vi "d(f4+g4u)_dx3.vi"(1 "x3_":dbl, 3 "x4_":dbl, 5 "F":dbl) -> (22 "d(f4+g4u)/dx3":dbl)   [LabVIEW 2014]
uses:
  <vilib>/Simulation/Implementation/Shared/SIMSCR Execution Mode.ctl
  <vilib>/Simulation/Scripting/Companion Diagram/SimConfigNode/SimParams.ctl
  <vilib>/Simulation/Scripting/Companion Diagram/SimConfigNode/_simSolvers.ctl
  <vilib>/Simulation/Param Hierarchy/Typedefs/SIMPH Param Control Actions.ctl
  <vilib>/Simulation/Implementation/Shared/NILVSim_ParamChanged.vi
  <vilib>/Simulation/Implementation/Shared/NILVSIM_BeginStep.vi
  <vilib>/Simulation/SignalArithmetic/Implementation/NILVSim Gain.llb/SIM Gain (scalar).vi
  <vilib>/Simulation/Implementation/Shared/NILVSim_Manager.vi
  <vilib>/Utility/error.llb/Clear Errors.vi
  <vilib>/Simulation/Implementation/Shared/NILVSim_FinalizeModel.vi
  <vilib>/Simulation/Implementation/Shared/SIM Unbundle Sim Info.vi
  <vilib>/Simulation/Implementation/Shared/SIMSH Read Queue.vi
  <vilib>/Simulation/Implementation/Shared/NILVSim_Initialize.vi
  <vilib>/Simulation/Utility/Implementation/NILVSim Get Time and IsAcceptedStep.vi
  <vilib>/Simulation/Implementation/Shared/NILVSim_GetModelError.vi
  <vilib>/Simulation/Implementation/Shared/SIM SimErrorHandler.vi
  <vilib>/Simulation/Implementation/Shared/SIM Bundle Sim Info.vi
  <vilib>/Simulation/Scripting/Companion Diagram/SimConfigNode/SimDog.xnode
  <vilib>/Simulation/Implementation/XNodeFramework/SimXNode/SimX.xnode
  <vilib>/Simulation/Implementation/Shared/NI_SIM_Implementation.lvlib
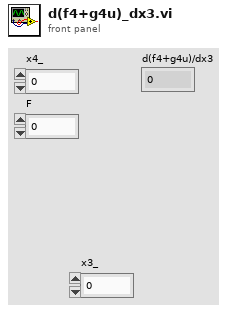
[diagram p1: front panel]
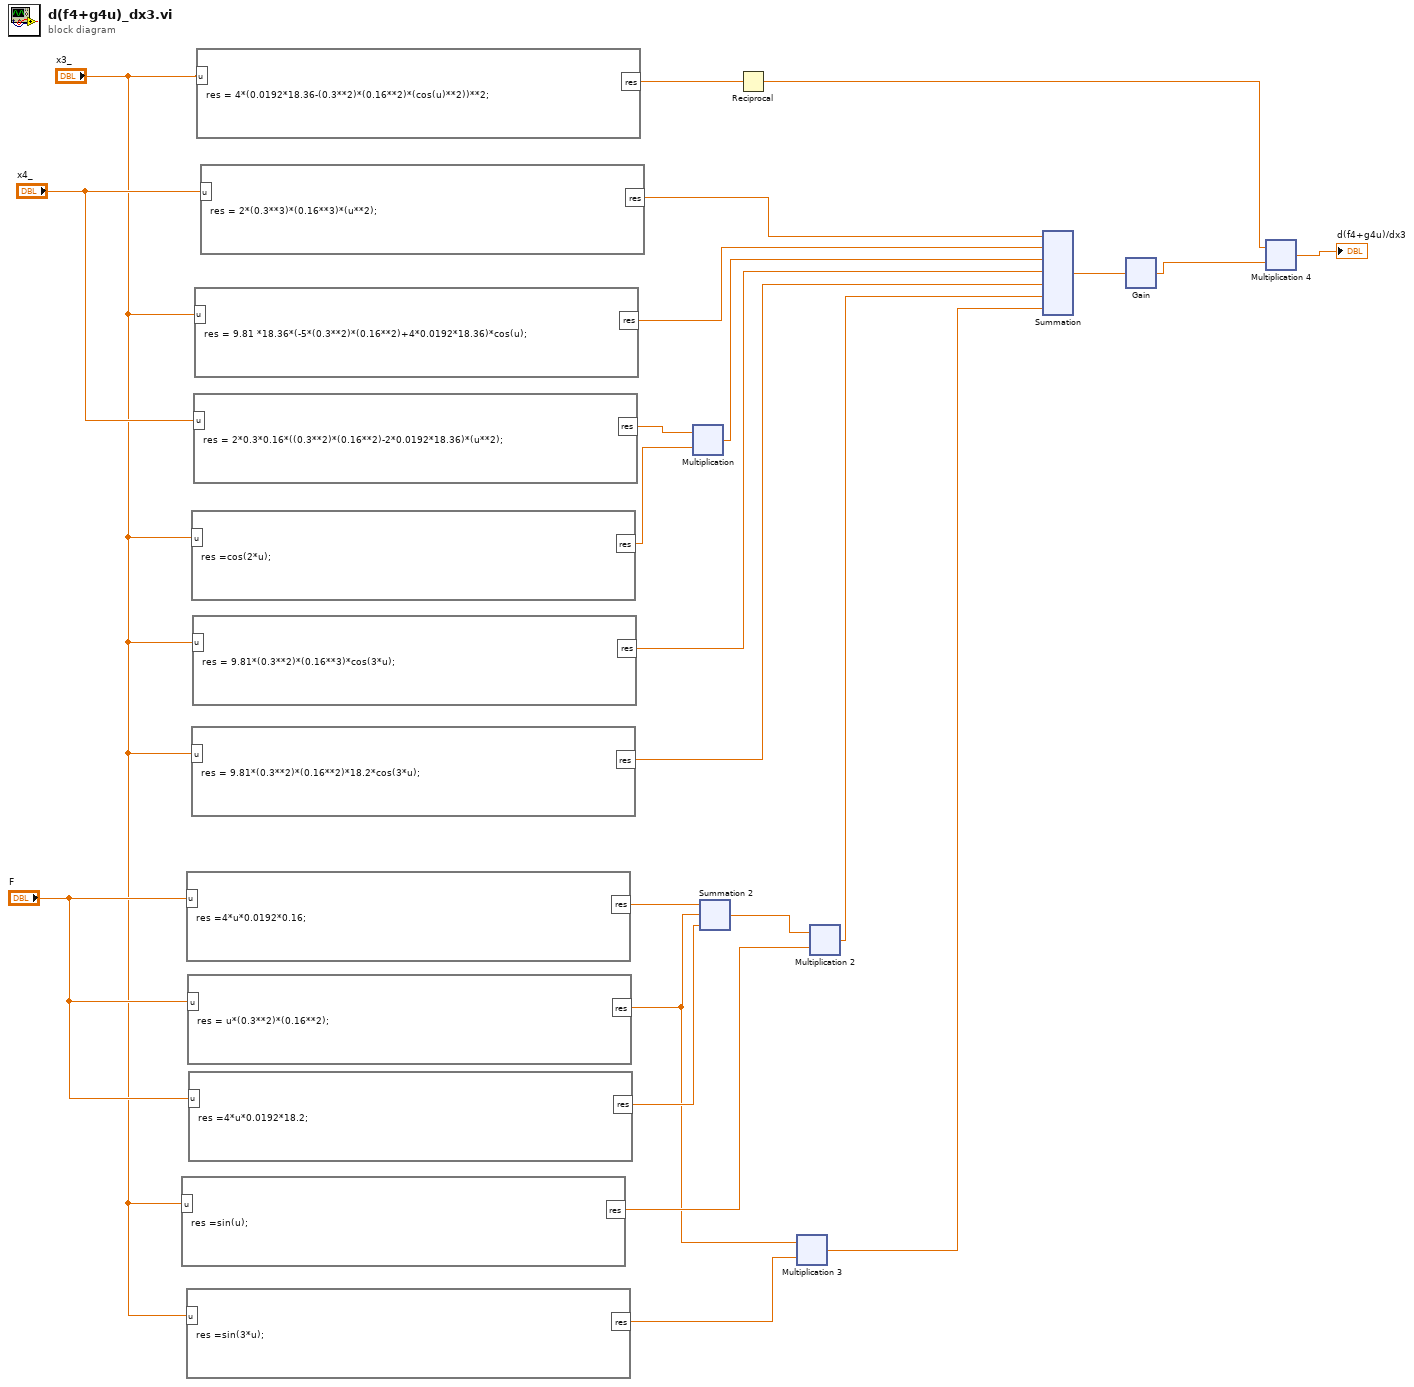
[diagram p0: block diagram]
diagram:
  n1 = formula code="res =sin(u);" ("Formelknoten 3")("u"="x3_") -> ("res"=w9:dbl)
  n2 = formula code="res =4*u*0.0192*0.16;" ("Formelknoten 6")("u"="F") -> ("res"=w14:dbl)
  n3 = formula code="res =sin(3*u);" ("Formelknoten 12")("u"="x3_") -> ("res"=w7:dbl)
  n4 = formula code="res = u*(0.3**2)*(0.16**2);" ("Formelknoten 5")("u"="F") -> ("res"=w8:dbl)
  n5 = formula code="res =4*u*0.0192*18.2;" ("Formelknoten 4")("u"="F") -> ("res"=w12:dbl)
  n6 = formula code="res =cos(2*u);" ("Formelknoten 9")("u"="x3_") -> ("res"=w18:dbl)
  n7 = formula code="res = 9.81*(0.3**2)*(0.16**2)*18.2*cos(3*u);" ("Formelknoten 7")("u"="x3_") -> ("res"=w15:dbl)
  n8 = formula code="res = 9.81*(0.3**2)*(0.16**3)*cos(3*u);" ("Formelknoten 8")("u"="x3_") -> ("res"=w16:dbl)
  n9 = formula code="res = 2*0.3*0.16*((0.3**2)*(0.16**2)-2*0.0192*18.36)*(u**2);" ("Formelknoten 10")("u"="x4_") -> ("res"=w19:dbl)
  n10 = formula code="res = 9.81 *18.36*(-5*(0.3**2)*(0.16**2)+4*0.0192*18.36)*cos(u);" ("Formelknoten 11")("u"="x3_") -> ("res"=w21:dbl)
  n11 = formula code="res = 4*(0.0192*18.36-(0.3**2)*(0.16**2)*(cos(u)**2))**2;" ("Formelknoten")("u"="x3_") -> ("res"=w23:dbl)
  n12 = formula code="res = 2*(0.3**3)*(0.16**3)*(u**2);" ("Formelknoten 2")("u"="x4_") -> ("res"=w22:dbl)
  n13 = xnode ("Multiplication")("Operand1"=w19, "Operand2"=w18) -> ("Result"=w17:dbl)
  n14 = xnode ("Summation 2")("Operand1"=w14, "Operand2"=w8, "Operand3"=w12) -> ("Result"=w10:dbl)
  n15 = Reciprocal ("Kehrwert")(x=w23) -> (1/x=w2:dbl)
  n16 = xnode ("Multiplication 3")("Operand1"=w8, "Operand2"=w7) -> ("Result"=w5:dbl)
  n17 = xnode ("Multiplication 2")("Operand1"=w10, "Operand2"=w9) -> ("Result"=w6:dbl)
  n18 = xnode ("Summation")("Operand1"=w22, "Operand2"=w21, "Operand3"=w17, "Operand4"=w16, "Operand5"=w15, "Operand6"=w6, "Operand7"=w5) -> ("Result"=w4:dbl)
  n19 = xnode "Gain"("input"=w4) -> ("output"=w3:dbl)  [unwired: 3 in]
  n20 = xnode ("Multiplication 4")("Operand1"=w2, "Operand2"=w3) -> ("Result"=→"d(f4+g4u)/dx3":dbl)
